vi "QDMH DequeueParse.vi"(8 "error in (no error)":errorcluster, 9 "Timeout":i32, 11 "queue":refnum<queue>) -> (0 "error out":errorcluster, 1 "Variant Data":variant, 2 "State":string, 3 "queue out":refnum<queue>)   [LabVIEW 2011]
doc: "This VI will parse a command from the data variant and will return both paramenters. It could be modified for futher functionality.\n\nAAL 9/09"
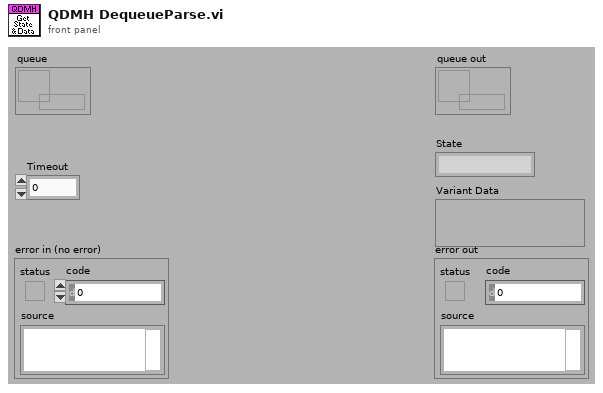
[diagram p1: front panel]
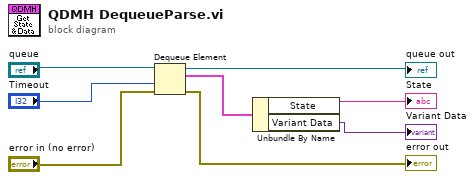
[diagram p0: block diagram]
diagram:
  n1 = Dequeue Element(queue="queue", timeout in ms (-1)="Timeout", error in (no error)="error in (no error)") -> (queue out=→"queue out":refnum<queue>, element=w3:cluster{"State":string, "Variant Data":variant}, error out=→"error out":errorcluster)  [unwired: 1 out]
  n2 = Unbundle By Name(w3) -> ("State"=→"State":string, "Variant Data"=→"Variant Data":variant)
